vi "Diagram.vi"(11 "Events":T1) -> ()   [LabVIEW 2023, in "SFC.lvlib"]
uses:
  SFC.lvlib
  TypeDef/Events TypeDef.ctl
panel:
  out "Queue Timeout":bool
  in  "Start":bool
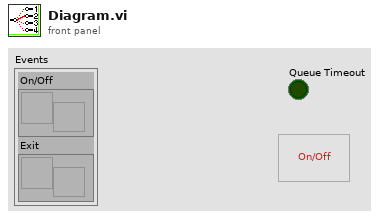
[diagram p1: front panel]
types:
  T1 = typedef "SFC.lvlib/Events TypeDef.ctl" = cluster{"On/Off":refnum<user-event>, "Exit":refnum<user-event>}
  T2 = typedef "SFC.lvlib/Control TypeDef.ctl" = cluster{"queue":refnum<queue>, "error":errorcluster, "Step":T3, "Algorythm":T3[]}
  T3 = typedef "SFC.lvlib/Step TypeDef.ctl" = cluster{"Name":string, "Timeout":dbl}
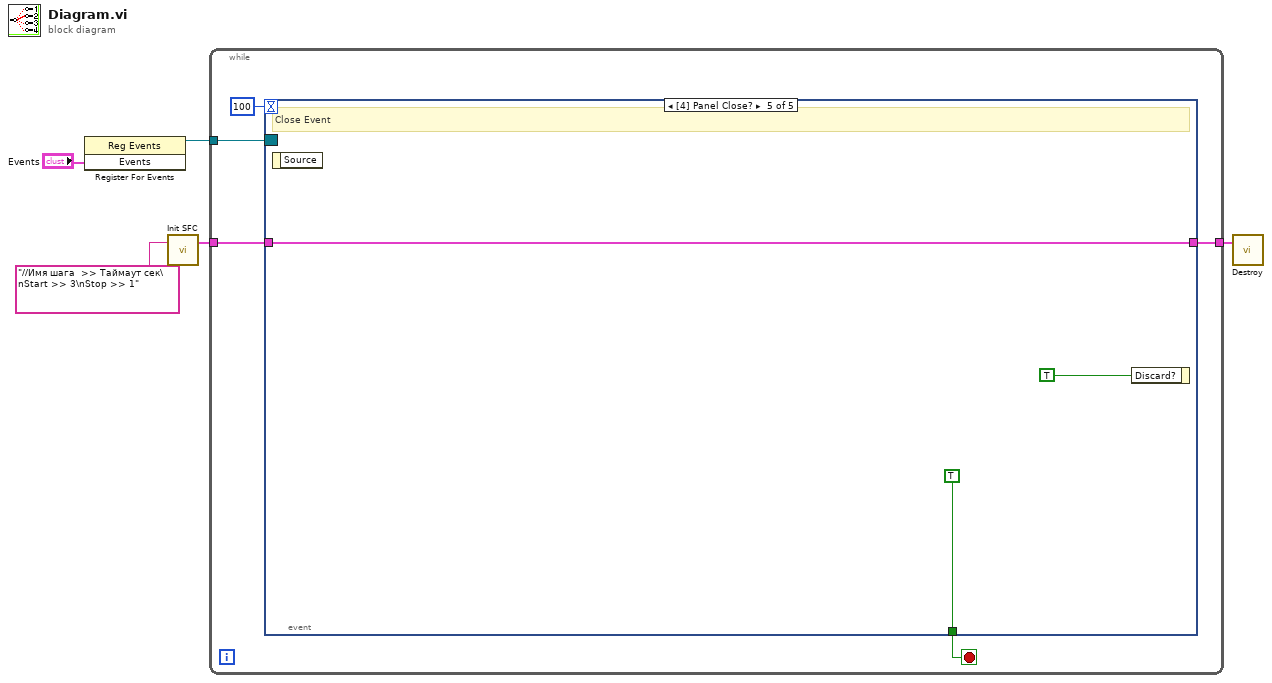
[diagram p0: block diagram]
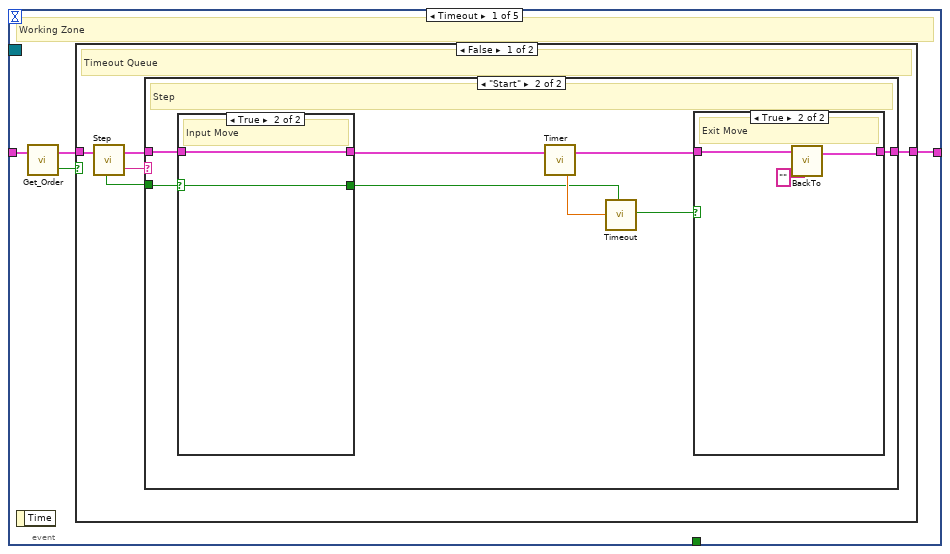
[diagram p2: hidden frame]
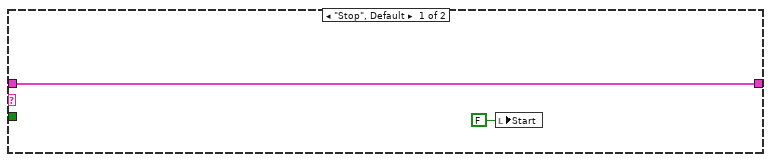
[diagram p3: hidden frame]
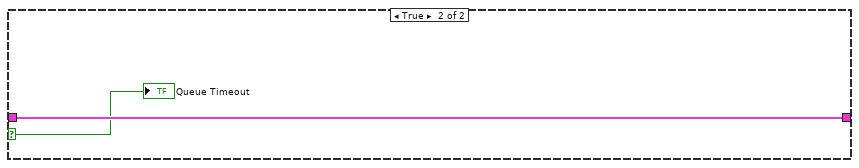
[diagram p6: hidden frame]
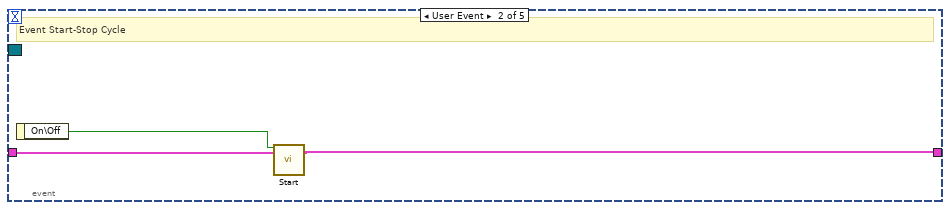
[diagram p7: hidden frame]
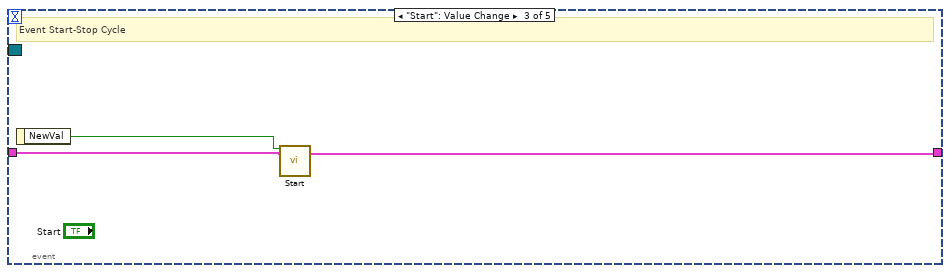
[diagram p8: hidden frame]
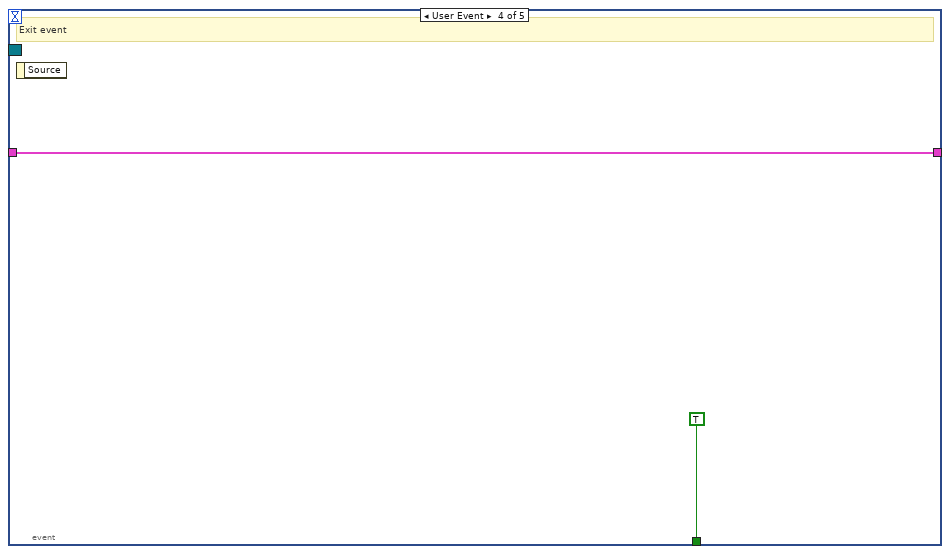
[diagram p9: hidden frame]
diagram:
  n1 = register-events("Events") -> (reference out=w5:refnum<event-registration>)  [unwired: 2 in, 1 out]
  n2 = call "Init SFC.vi"("Algo"="//Имя шага  >> Таймаут сек\nStart >> 3\nStop >> 1") -> ("Control"=w3:T2)  [unwired: 18 in]
  n3 = while {
    tunnel: w5 -> [w10]
    tunnel: w3 -> [w9]
    tunnel: [w8] -> w2
    stop <- w6 stop-if-true
    n4 = event shown="[4] Panel Close?" {
      selector: w10 -> [_ _ _ _ _]
      dyn-events: _ -> [_ _ _ _ _]
      timeout: 100 -> [_ _ _ _ _]
      tunnel: w9 -> [w13 w42 w45 w47 w48]
      tunnel: [w14 w41 w43 w47 w48] -> w8
      tunnel: [_ _ _ TRUE TRUE] -> w6
      event Timeout {
        # "Working Zone"
        n5 = event-data() -> ()  [unwired: 1 in, 1 out]
        n6 = call "Get_Order.vi"("Control in"=w13) -> ("timed out?"=w11:bool, "Control out"=w12:T2)  [unwired: 17 in]
        n7 = case shown="False" w11 {
          selector: w11 -> [_ w38]
          tunnel: w12 -> [w18 w39]
          tunnel: [w19 w39] -> w14
          frame False {
            # "Timeout Queue"
            n8 = call "Step.vi"("Control in"=w18) -> ("Init?"=w15:bool, "Name"=w16:string, "Control out"=w17:T2)  [unwired: 16 in]
            n9 = case shown="\"Start\"" w16 {
              tunnel: w17 -> [w21 w28]
              tunnel: w15 -> [_ w29]
              tunnel: [w21 w27] -> w19
              frame "Stop", Default {
                n10 = local write "Start"(FALSE ("Start")) -> ()
              }
              frame "Start" {
                # "Step"
                n11 = case shown="True" w29 {
                  selector: w29 -> [w34 w36]
                  tunnel: [w35 w37] -> w24
                  tunnel: w28 -> [w35 w37]
                  tunnel: [w34 w36] -> w22
                  frame False {
                  }
                  frame True {
                    # "Input Move"
                  }
                }
                n12 = call "Timer.vi"("Control in"=w24) -> ("Timeout"=w23:dbl, "Control out"=w25:T2)  [unwired: 17 in]
                n13 = call "Timeout.vi"("Timeout"=w23, "RST"=w22) -> ("Done"=w26:bool)  [unwired: 16 in, 1 out]
                n14 = case shown="True" w26 {
                  tunnel: [w30 w32] -> w27
                  tunnel: w25 -> [w30 w33]
                  frame False {
                  }
                  frame True {
                    # "Exit Move"
                    n15 = call "BackTo.vi"("Control in"=w33, "Back Step?"="" ("Step")) -> ("Control out"=w32:T2)  [unwired: 17 in]
                  }
                }
              }
            }
          }
          frame True {
            "Queue Timeout" <- w38
          }
        }
      }
      event User Event {
        # "Event Start-Stop Cycle"
        n16 = event-data() -> ("On\\Off"=w40:bool)  [unwired: 1 in]
        n17 = call "Start.vi"("On/Off"=w40, "Control in"=w42) -> ("Control out"=w41:T2)  [unwired: 17 in]
      }
      event "Start": Value Change {
        # "Event Start-Stop Cycle"
        n18 = event-data() -> ("NewVal"=w44:bool)  [unwired: 1 in]
        n19 = call "Start.vi"("On/Off"=w44, "Control in"=w45) -> ("Control out"=w43:T2)  [unwired: 17 in]
      }
      event User Event {
        # "Exit event"
        n20 = event-data() -> ()  [unwired: 1 in, 1 out]
      }
      event Panel Close? {
        # "Close Event"
        n21 = event-data() -> ()  [unwired: 1 in, 1 out]
        n22 = event-data("Discard?"=TRUE) -> ()  [unwired: 1 in, 1 out]
      }
    }
  }
  n23 = call "Destroy.vi"("Control"=w2) -> ()  [unwired: 19 in]
